vi "NeedRecalcPath.vi"(4 "SmoothPath":dbl[][](array[numeric]), 5 "Initial State":dbl[](array[numeric]), 7 "Pos x,y":dbl[](array[numeric]), 9 "IA State":T1={"our_robots"=[], "enemy_robots"=[], "balls"=[], "geometry"={"line_width"=0, "field_length"=0, "field_width"=0, "boundary_width"=0, "referee_width"=0, "goal_width"=0, "goal_depth"=0, "goal_wall_width"=0, "center_circle_radius"=0, "defense_radius"=0, "defense_stretch"=0, "free_kick_from_defense_dist"=0, "penalty_spot_from_field_line_dist"=0, "penalty_line_from_spot_dist"=0}, "IA Judge"={"stage"="", "command"="", "our_goalie_id"=0.0, "enemy_goalie_id"=0.0, "command enum"=enum."Halt", "Time"=enum."Azul"}, "Received Timestamp"=timestamp(0 s since 1904-01-01), "Events"={"Touch"=FALSE, "Ball out"=FALSE, "id touch"=0.0, "Ball out of \nVision"=FALSE, "Ball inside \nGoalie area"=FALSE, "Robot not responding"=FALSE, "Robots responding status"=[1.0, 1.0, 1.0, 1.0, 1.0, 1.0], "Enemy Ball \nPossession"=FALSE, "Pass State"=FALSE, "id end of pass"=0.0, "Kick"=FALSE, "Id ini Possession"=0.0, "Ball Possesion"=FALSE, "Id Possesion"=0.0}}, 10 "Robot":T2, 11 "Dest x,y":dbl[](array[numeric])) -> (3 "NeedRecalc":bool)   [LabVIEW 2017]
uses:
  Core/AI Robot.ctl
  Intel/Functions Enum.ctl
  Intel/AttackerStates.ctl
  PathDests.ctl
  PathDest.ctl
  Core/AI Input.ctl
  Core/AI Ball.ctl
  Core/Field Size.ctl
  Core/AI Judge.ctl
  Intel/Command Enum.ctl
  Util/Events/Events.ctl
  <vilib>/Analysis/_algsub.llb/Real Vector Norm.vi
  <vilib>/Analysis/NI_AALPro.lvlib
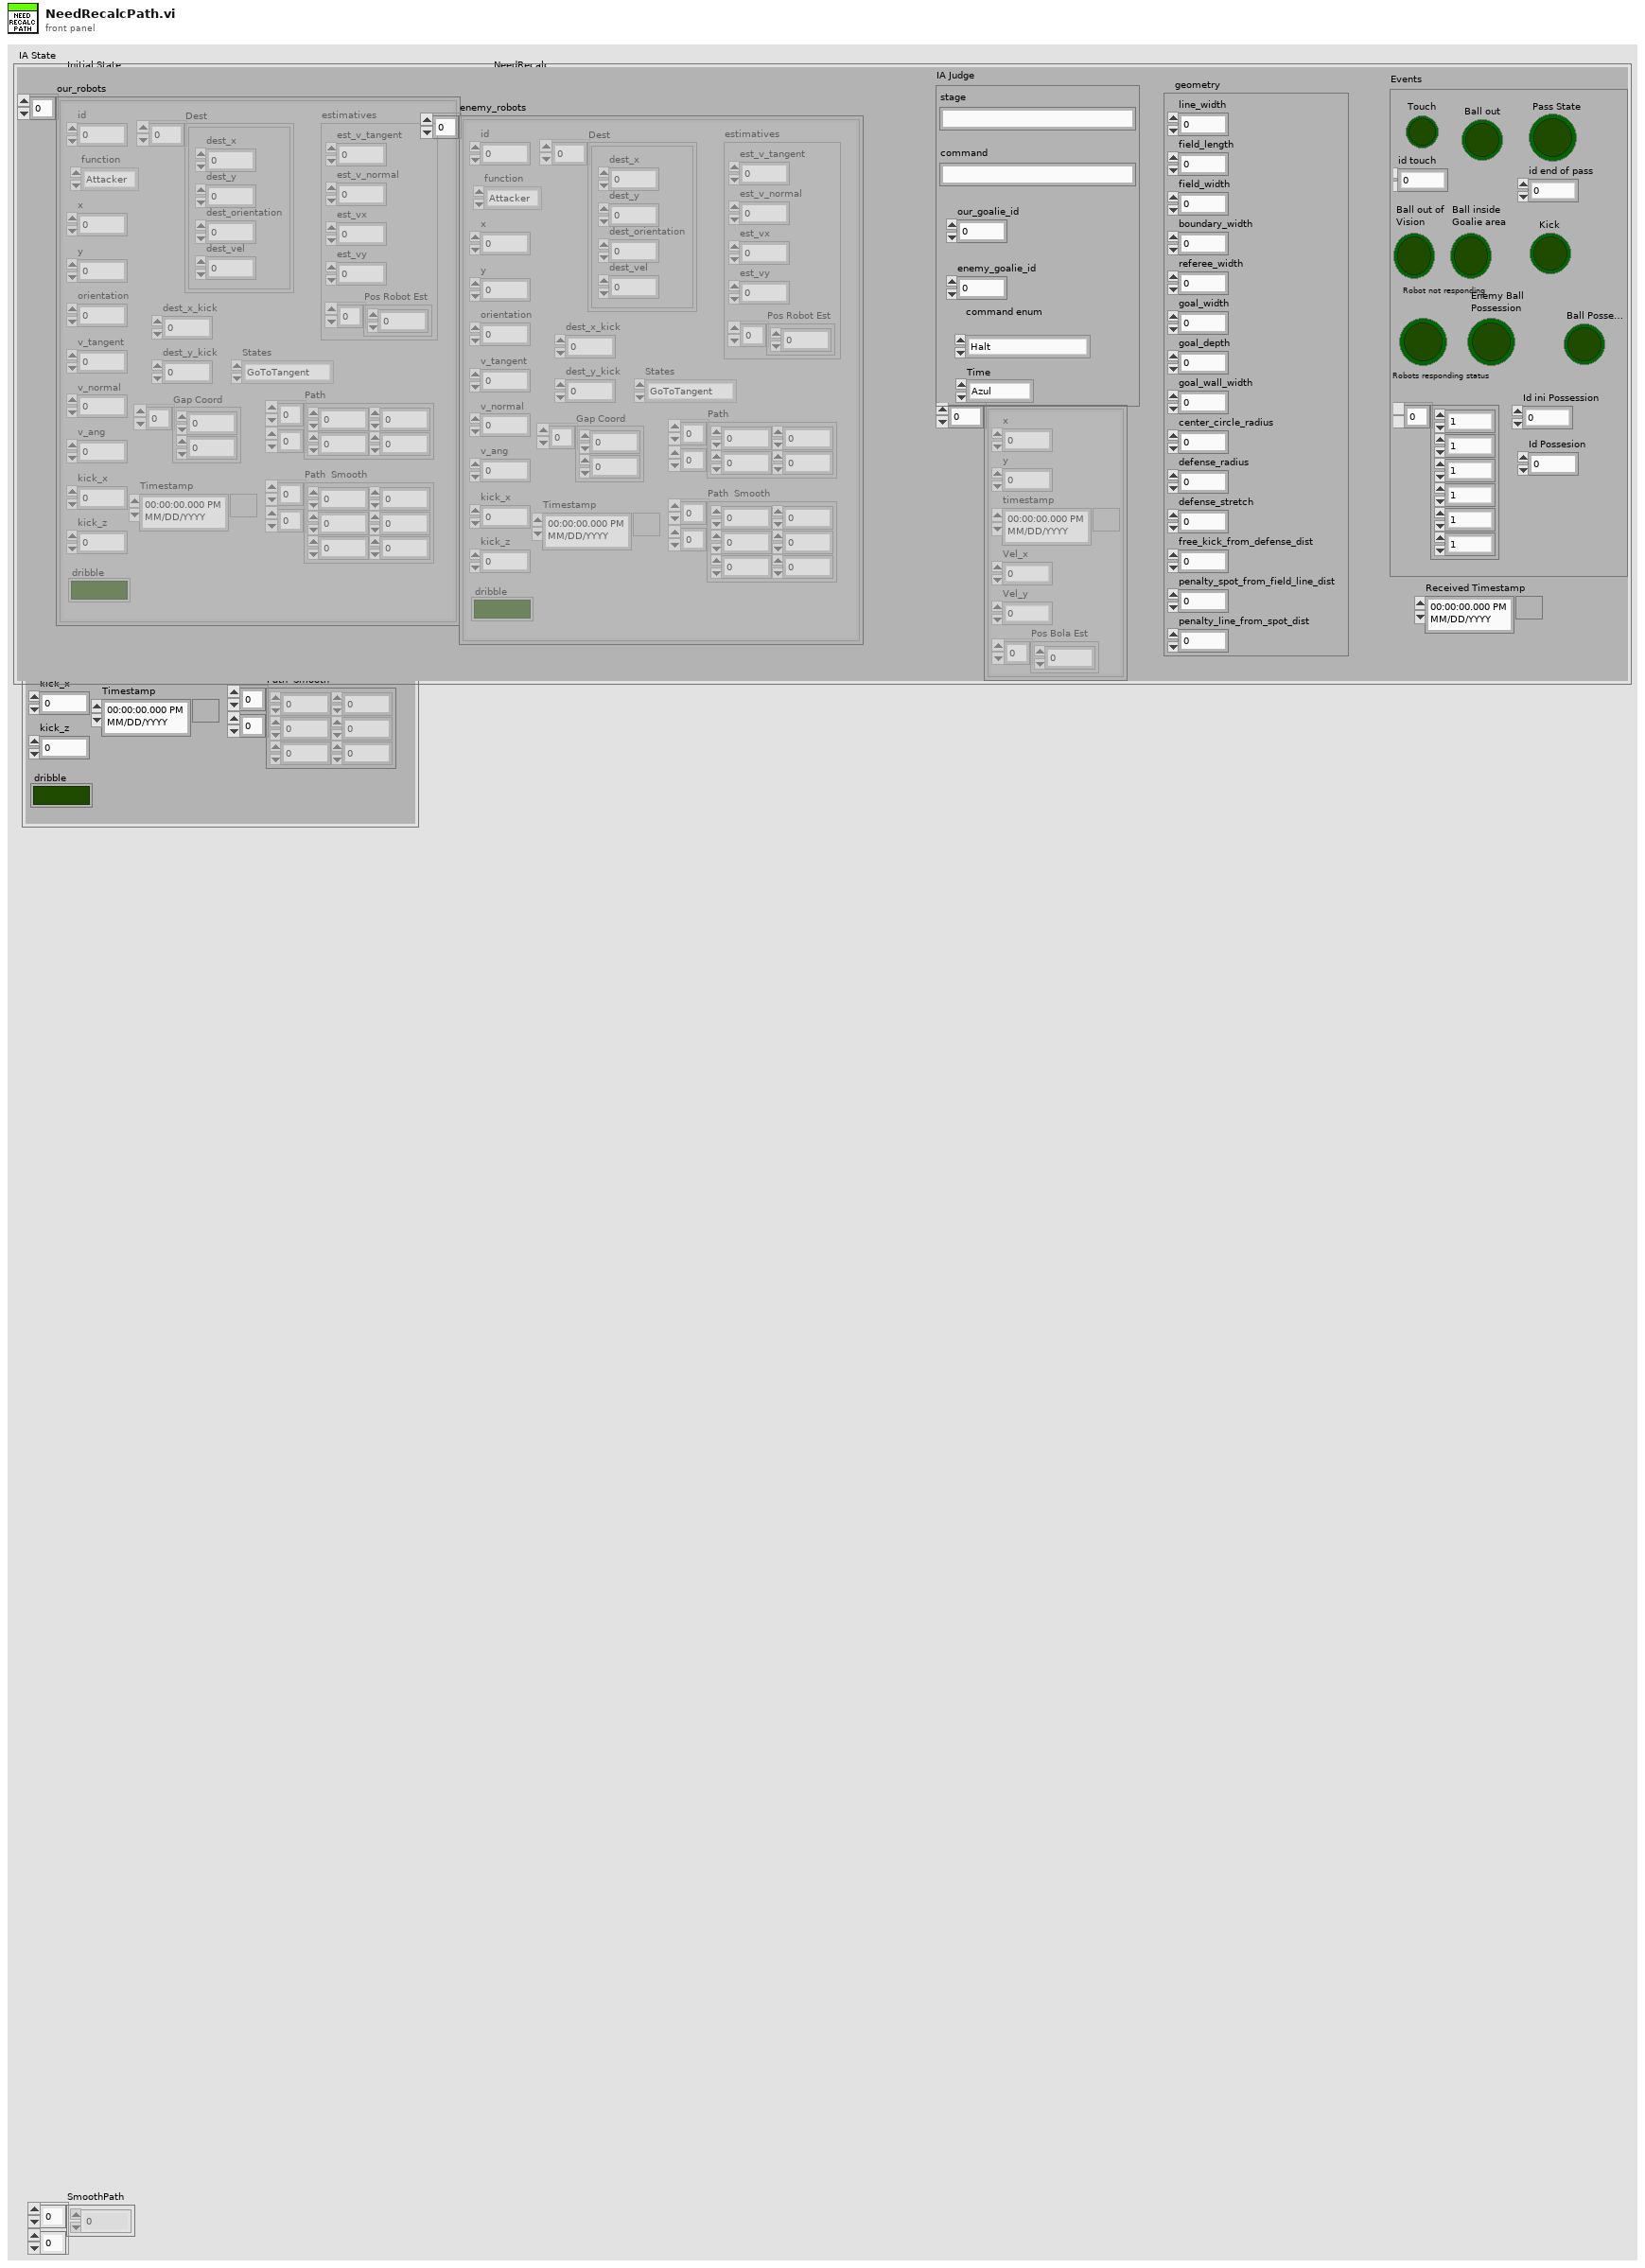
[diagram p1: front panel]
types:
  T1 = typedef "AI Input.ctl" = cluster{"our_robots":T2[], "enemy_robots":T2[], "balls":T7[], "geometry":T8, "IA Judge":T9, "Received Timestamp":timestamp, "Events":T11}
  T2 = typedef "AI Robot.ctl" = cluster{"id":u32, "function":T3, "x":dbl, "y":dbl, "orientation":dbl, "v_tangent":dbl, "v_normal":dbl, "v_ang":dbl, "kick_x":dbl, "kick_z":dbl, "dribble":bool, "Timestamp":timestamp, "estimatives":cluster{"est_v_tangent":dbl, "est_v_normal":dbl, "est_vx":dbl, "est_vy":dbl, "Pos Robot Est":dbl[]}, "dest_x_kick":dbl, "dest_y_kick":dbl, "Gap Coord":dbl[], "States":T4, "Path ":dbl[][], "Path  Smooth":dbl[][], "Dest":T5}
  T3 = typedef "Functions Enum.ctl" = enum16{"Attacker", "Goalie", "Defender", "Striker", "Goto 0", "Dummy", "Kicker", "ZigZag"}
  T4 = typedef "AttackerStates.ctl" = enum16{"Pass", "GoToTangent", "BallGetting", "GoToKick", ""}
  T5 = typedef "PathDests.ctl" = T6[]
  T6 = typedef "PathDest.ctl" = cluster{"dest_x":dbl, "dest_y":dbl, "dest_orientation":dbl, "dest_vel":dbl}
  T7 = typedef "AI Ball.ctl" = cluster{"x":dbl, "y":dbl, "timestamp":timestamp, "Vel_x":dbl, "Vel_y":dbl, "Pos Bola Est":dbl[]}
  T8 = typedef "Field Size.ctl" = cluster{"line_width":u32, "field_length":u32, "field_width":u32, "boundary_width":u32, "referee_width":u32, "goal_width":u32, "goal_depth":u32, "goal_wall_width":u32, "center_circle_radius":u32, "defense_radius":u32, "defense_stretch":u32, "free_kick_from_defense_dist":u32, "penalty_spot_from_field_line_dist":u32, "penalty_line_from_spot_dist":u32}
  T9 = typedef "AI Judge.ctl" = cluster{"stage":string, "command":string, "our_goalie_id":dbl, "enemy_goalie_id":dbl, "command enum":T10, "Time":enum16{"Azul", "Amarelo"}}
  T10 = typedef "Command Enum.ctl" = enum16{"Halt", "Stop", "Force Start", "PKA Normal Start", "Prepare Kickoff Ally", "PKE Normal Start", "Prepare Kickoff Enemy", "Prepare Penalty Ally", "PPA Normal Start", "Prepare Penalty Enemy", "PPE Normal Start", "Direct Free Enemy", "Direct Free Ally", "Indirect Free Enemy", "Indirect Free Ally", "Timeout Enemy", "Timeout Ally", "Goal Enemy", "Goal Ally", "Ball Placement Enemy", "Ball Placement Ally", "Normal Half Time", "Extra Time Break", "Extra Half Time", "None", "Post Game"}
  T11 = typedef "Events.ctl" = cluster{"Touch":bool, "Ball out":bool, "id touch":dbl, "Ball out of \nVision":bool, "Ball inside \nGoalie area":bool, "Robot not responding":bool, "Robots responding status":dbl[], "Enemy Ball \nPossession":bool, "Pass State":bool, "id end of pass":dbl, "Kick":bool, "Id ini Possession":dbl, "Ball Possesion":bool, "Id Possesion":dbl}
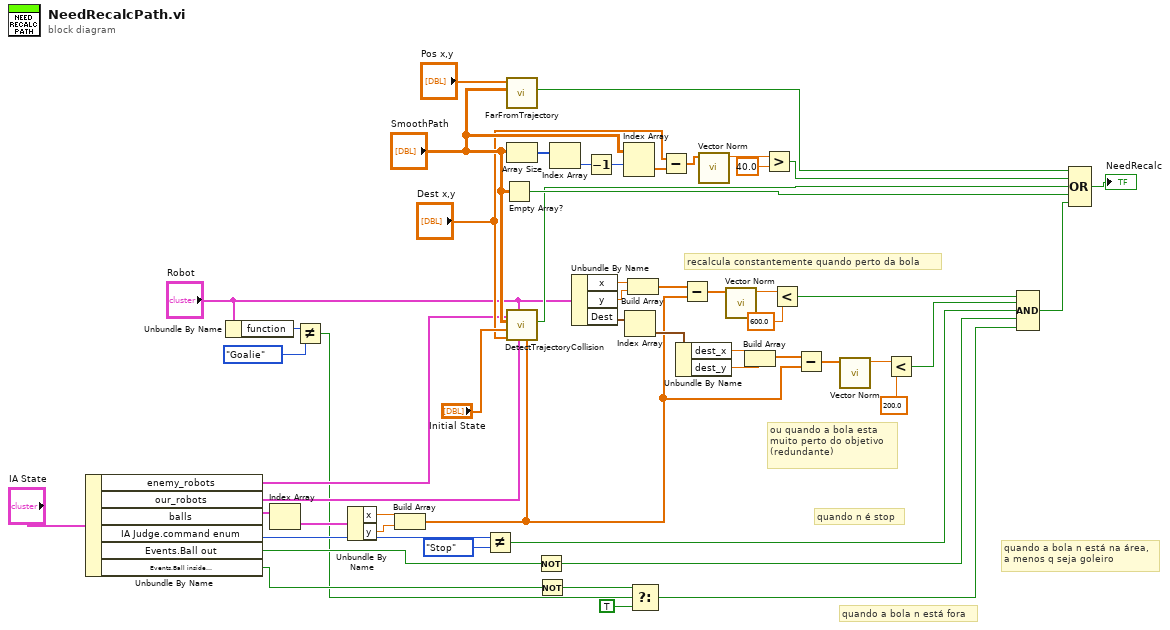
[diagram p0: block diagram]
diagram:
  # "ou quando a bola esta\nmuito perto do objetivo\n(redundante)"
  # "quando a bola n está na área,\na menos q seja goleiro"
  # "quando n é stop"
  # "quando a bola n está fora"
  # "recalcula constantemente quando perto da bola"
  n1 = Unbundle By Name("IA State") -> ("enemy_robots"=w37:T2[], "our_robots"=w36:T2[], "balls"=w35:T7[], "IA Judge.command enum"=w16:T10, "Events.Ball out"=w11:bool, "Events.Ball inside \nGoalie area"=w5:bool)
  n2 = Unbundle By Name("Robot") -> ("function"=w13:T3)
  n3 = Index Array(array=w35) -> (element=w34:T7)  [unwired: 1 in]
  n4 = Not Equal?(x=w13, y=Functions_Enum."Goalie") -> (x != y?=w3:bool)
  n5 = Unbundle By Name(w34) -> ("x"=w30:dbl, "y"=w29:dbl)
  n6 = Build Array(w30, w29) -> (w17:dbl[])
  n7 = Not Equal?(x=w16, y=Command_Enum."Stop") -> (x != y?=w7:bool)
  n8 = Empty Array?(array="SmoothPath") -> (empty?=w49:bool)
  n9 = call "FarFromTrajectory.vi"("Path"="SmoothPath", "Position"="Pos x,y") -> ("Far from trajectory?"=w51:bool)  [unwired: 9 in]
  n10 = Array Size(array="SmoothPath") -> (size(s)=w40:i32[])
  n11 = call "DetectTrajectoryCollision.vi"("ball"=w17, "our_robots"=w36, "Robot in"="Robot", "Goal"="Dest x,y", "Initial State"="Initial State", "Last Path"="SmoothPath", "enemy_robots"=w37) -> ("Collision"=w39:bool)  [unwired: 4 in]
  n12 = Not(x=w11) -> (.not. x?=w6:bool)
  n13 = Not(x=w5) -> (.not. x?=w4:bool)
  n14 = Index Array(array=w40) -> (element=w47:i32)  [unwired: 1 in]
  n15 = Unbundle By Name("Robot") -> ("x"=w33:dbl, "y"=w32:dbl, "Dest"=w26:T5)
  n16 = Decrement(x=w47) -> (x-1=w46:i32)
  n17 = Index Array(array="SmoothPath", index (row)=w46) -> (element=w41:dbl[])  [unwired: 1 in]
  n18 = Index Array(array=w26) -> (element=w25:T6)  [unwired: 1 in]
  n19 = Build Array(w33, w32) -> (w31:dbl[])
  n20 = Select(t=w4, s=w3, f=TRUE) -> (s? t:f=w1:bool)
  n21 = Subtract(x="Dest x,y", y=w41) -> (x-y=w42:dbl[])
  n22 = Unbundle By Name(w25) -> ("dest_x"=w23:dbl, "dest_y"=w22:dbl)
  n23 = Subtract(x=w31, y=w17) -> (x-y=w28:dbl[])
  n24 = call-poly <vilib>:"Vector Norm.vi"("Input Vector"=w42) -> ("norm"=w43:dbl)  [unwired: 9 in, 1 out]
  n25 = call-poly <vilib>:"Vector Norm.vi"("Input Vector"=w28) -> ("norm"=w27:dbl)  [unwired: 9 in, 1 out]
  n26 = Build Array(w23, w22) -> (w18:dbl[])
  n27 = Greater?(x=w43, y=40.0) -> (0:w44:bool)
  n28 = Less?(x=w27, y=600.0) -> (x < y?=w9:bool)
  n29 = Subtract(x=w18, y=w17) -> (x-y=w19:dbl[])
  n30 = call-poly <vilib>:"Vector Norm.vi"("Input Vector"=w19) -> ("norm"=w20:dbl)  [unwired: 9 in, 1 out]
  n31 = Less?(x=w20, y=200.0) -> (x < y?=w8:bool)
  n32 = Compound Arithmetic op=AND(w9, w8, w7, w6, w1) -> (w10:bool)
  n33 = Compound Arithmetic op=OR(w51, w44, w39, w49, w10) -> (→"NeedRecalc":bool)
